vi "for con condicional.vi"() -> ()   [LabVIEW 2020]
panel:
  out "x*y":dbl
  out "Numeric 2":i32
  in  "Numeric":i32
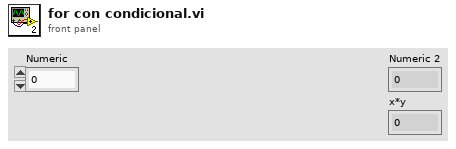
[diagram p1: front panel]
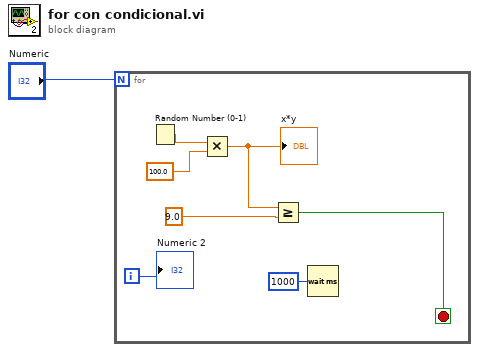
[diagram p0: block diagram]
diagram:
  n1 = for {
    N: "Numeric" -> [_]
    i -> [w8]
    stop <- w2 stop-if-true
    n2 = Random Number (0-1)() -> (number: 0 to 1=w6:dbl)
    n3 = Multiply(x=w6, y=100.0) -> (x*y=w5:dbl)
    "x*y" <- w5
    n4 = Greater Or Equal?(x=w5, y=9.0) -> (x >= y?=w2:bool)
    n5 = Wait (ms)(milliseconds to wait=u32 1000) -> ()  [unwired: 1 out]
    "Numeric 2" <- w8
  }
